vi "CalcRatios.vi"(9 "Run Summary":T2) -> (1 "Run Ratios":T1)   [LabVIEW 2011]
panel:
  in  "Run Ratios In":T1
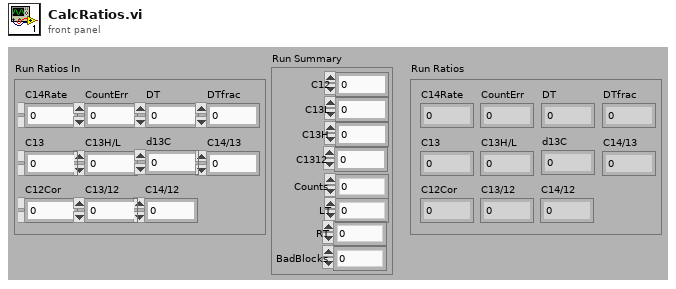
[diagram p1: front panel]
types:
  T1 = cluster{"C14Rate":dbl, "CountErr":dbl, "DT":dbl, "DTfrac":dbl, "C13":dbl, "C13H/L":dbl, "d13C":dbl, "C14/13":dbl, "C12Cor":dbl, "C13/12":dbl, "C14/12":dbl}
  T2 = cluster{"C12":dbl, "C13L":dbl, "C13H":dbl, "Counts":u32, "LT":dbl, "RT":dbl, "BadBlocks":u8, "C1312":dbl}
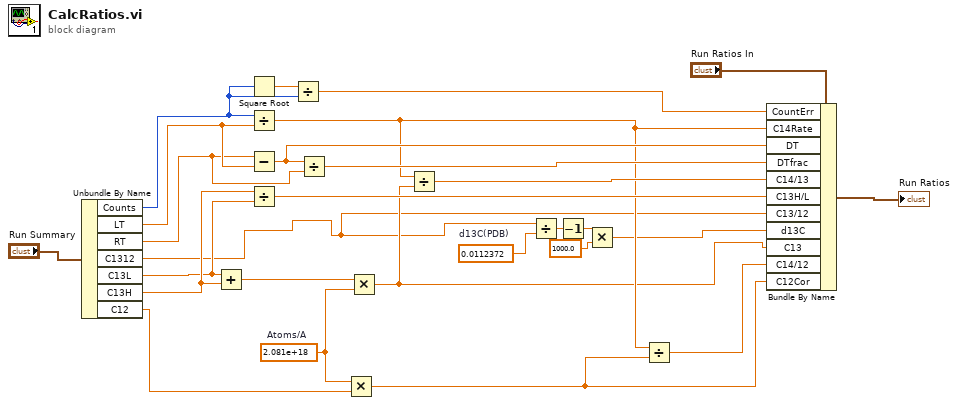
[diagram p0: block diagram]
diagram:
  w22 = 0.0112372  # d13C(PDB)
  w21 = 2.081e+18  # Atoms/A
  n1 = Unbundle By Name("Run Summary") -> ("Counts"=w16:u32, "LT"=w19:dbl, "RT"=w18:dbl, "C1312"=w2:dbl, "C13L"=w3:dbl, "C13H"=w17:dbl, "C12"=w1:dbl)
  n2 = Add(x=w3, y=w17) -> (x+y=w27:dbl)
  n3 = Square Root(x=w16) -> (sqrt(x)=w26:dbl)
  n4 = Divide(x=w16, y=w19) -> (x/y=w9:dbl)
  n5 = Subtract(x=w18, y=w19) -> (x-y=w13:dbl)
  n6 = Divide(x=w17, y=w3) -> (x/y=w10:dbl)
  n7 = Divide(x=w26, y=w16) -> (x/y=w8:dbl)
  n8 = Divide(x=w13, y=w18) -> (x/y=w12:dbl)
  n9 = Multiply(x=w21, y=w1) -> (x*y=w6:dbl)
  n10 = Multiply(x=w27, y=w21) -> (x*y=w5:dbl)
  n11 = Divide(x=w9, y=w5) -> (x/y=w11:dbl)
  n12 = Divide(x=w2, y=w22) -> (x/y=w24:dbl)
  n13 = Decrement(x=w24) -> (x-1=w25:dbl)
  n14 = Multiply(x=w25, y=1000.0) -> (x*y=w4:dbl)
  n15 = Divide(x=w9, y=w6) -> (x/y=w7:dbl)
  n16 = Bundle By Name(cluster="Run Ratios In", "CountErr"=w8, "C14Rate"=w9, "DT"=w13, "DTfrac"=w12, "C14/13"=w11, "C13H/L"=w10, "C13/12"=w2, "d13C"=w4, "C13"=w5, "C14/12"=w7, "C12Cor"=w6) -> (→"Run Ratios":T1)
